vi "Remove_underscores_at_ends.vi"(1 "String in":string) -> (0 "String out":string)   [LabVIEW 2011]
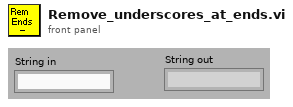
[diagram p1: front panel]
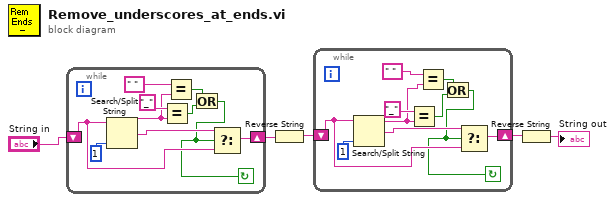
[diagram p0: block diagram]
diagram:
  n1 = while {
    shift-left: "String in" -> [w12]
    shift-right: [w11] -> w1
    stop <- w6 continue-if-true
    n2 = Search/Split String(string=w12, offset (0)=1 ("length")) -> (substring before match=w10:string, match + rest of string=w13:string)  [unwired: 2 out]
    n3 = Equal?(x="_", y=w10) -> (x = y?=w8:bool)
    n4 = Equal?(x=" ", y=w10) -> (x = y?=w7:bool)
    n5 = Or(x=w7, y=w8) -> (x .or. y?=w6:bool)
    n6 = Select(t=w13, s=w6, f=w12) -> (s? t:f=w11:string)
  }
  n7 = Reverse String(1:w1) -> (0:w2:string)
  n8 = while {
    shift-left: w2 -> [w22]
    shift-right: [w21] -> w3
    stop <- w16 continue-if-true
    n9 = Search/Split String(string=w22, offset (0)=1 ("length")) -> (substring before match=w18:string, match + rest of string=w23:string)  [unwired: 2 out]
    n10 = Equal?(x="_", y=w18) -> (x = y?=w17:bool)
    n11 = Equal?(x=" ", y=w18) -> (x = y?=w20:bool)
    n12 = Or(x=w20, y=w17) -> (x .or. y?=w16:bool)
    n13 = Select(t=w23, s=w16, f=w22) -> (s? t:f=w21:string)
  }
  n14 = Reverse String(1:w3) -> (0:→"String out":string)
